vi "Set Up Dialog - Circulation Lab.vi"() -> ()   [LabVIEW 2012]
panel:
  out "Set Up Instructions":string="This lab uses both the Blood Pressue and Pulse sensors. Click the buttons below to learn how to set up each sensor. Be sure to connect the Pulse sensor to channel 1 and the blood pressure sensor to channel 2."
  in  "PTN Set Up":bool
  in  "BP Set Up":bool
  # "Circulation Lab - Set Up"
  # "Blood Pressure Sensor"
  # "Pulse Sensor (PTN - 104)"
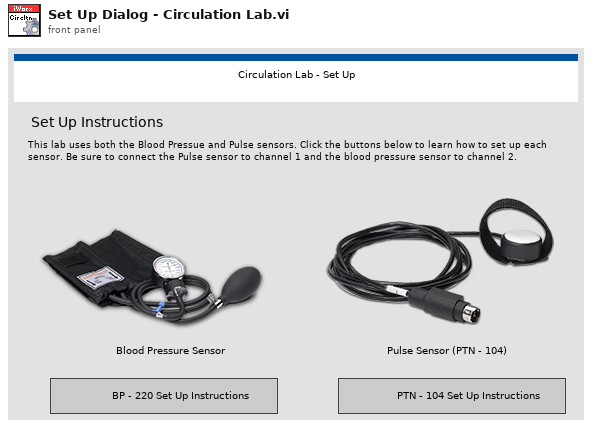
[diagram p1: front panel]
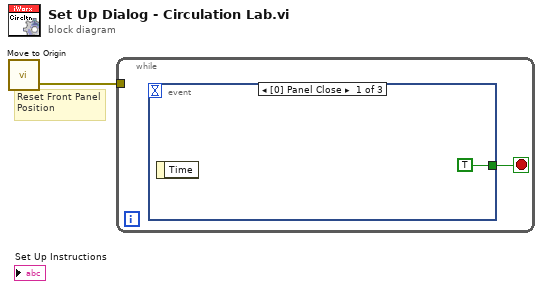
[diagram p0: block diagram]
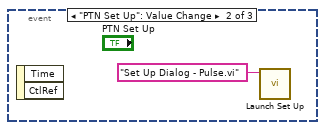
[diagram p2: hidden frame]
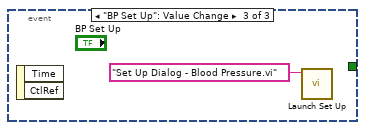
[diagram p3: hidden frame]
diagram:
  # "Reset Front Panel Position"
  n1 = call "Move to Origin.vi"() -> ("Error Out"=w1:errorcluster)  [unwired: 3 in]
  n2 = while {
    tunnel: w1 -> [_]
    stop <- w2 stop-if-true
    n3 = event shown="[0] Panel Close" {
      selector: _ -> [_ _ _]
      dyn-events: _ -> [_ _ _]
      timeout: _ -> [_ _ _]
      tunnel: [TRUE _ _] -> w2
      event Panel Close {
        n4 = event-data() -> ()  [unwired: 1 in, 1 out]
      }
      event "PTN Set Up": Value Change {
        n5 = event-data() -> ()  [unwired: 1 in, 2 out]
        n6 = call "Launch Set Up.vi"("name or relative path"="Set Up Dialog - Pulse.vi") -> ()  [unwired: 9 in, 2 out]
      }
      event "BP Set Up": Value Change {
        n7 = event-data() -> ()  [unwired: 1 in, 2 out]
        n8 = call "Launch Set Up.vi"("name or relative path"="Set Up Dialog - Blood Pressure.vi") -> ()  [unwired: 9 in, 2 out]
      }
    }
  }
